vi "test Can Retry A Timed Out Future.vi"(8 "error in (no error)":errorcluster, 11 "TestCase in":refnum<class "Futures Tests.lvclass">) -> (0 "error out":errorcluster, 3 "TestCase out":refnum<class "Futures Tests.lvclass">)   [LabVIEW 2017, in "Futures Tests.lvclass"]
uses:
  Futures Tests.lvclass
  <vilib>/addons/_JKI Toolkits/VI Tester/TestCase.llb/TestCase.lvclass
  Futures/Futures.lvlib
  Futures/Future/Future.lvclass
  Futures/Promise/Promise.lvclass
  C:/Program Files (x86)/National Instruments/LabVIEW 2017/vi.lib/addons/_JKI Toolkits/VI Tester/TestCase.llb/TestCase.lvclass
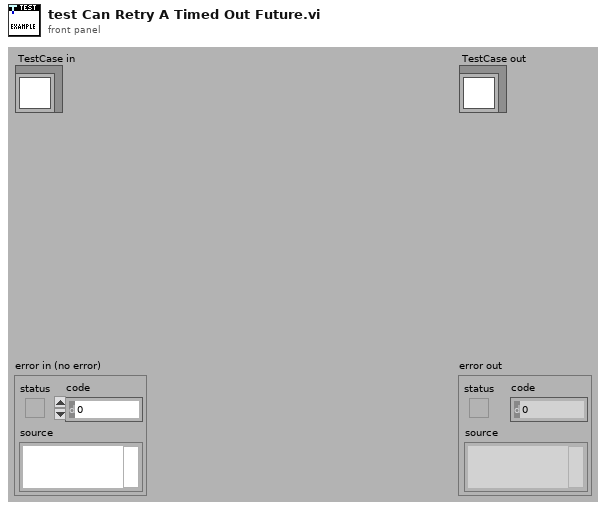
[diagram p1: front panel]
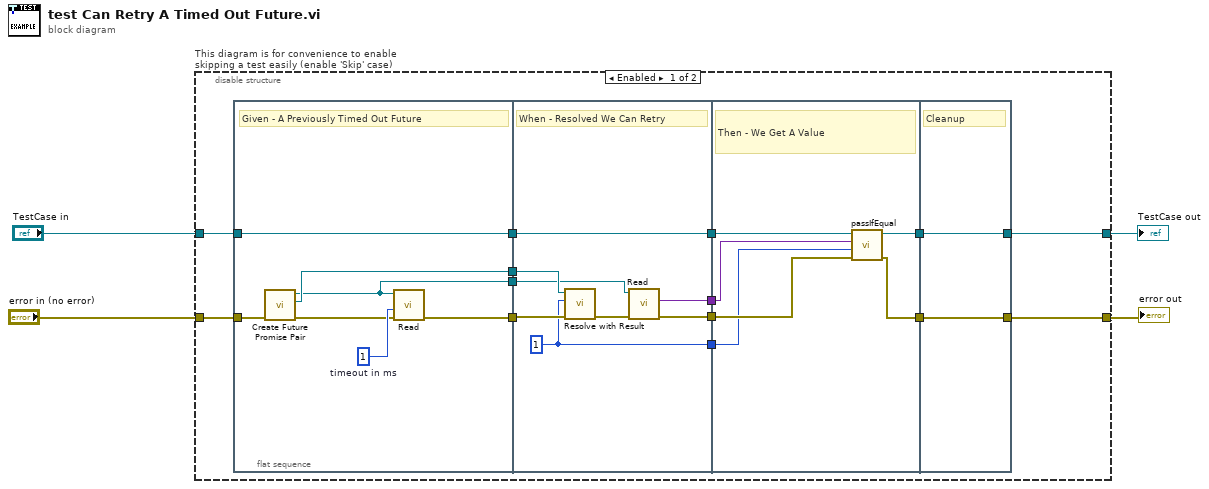
[diagram p0: block diagram]
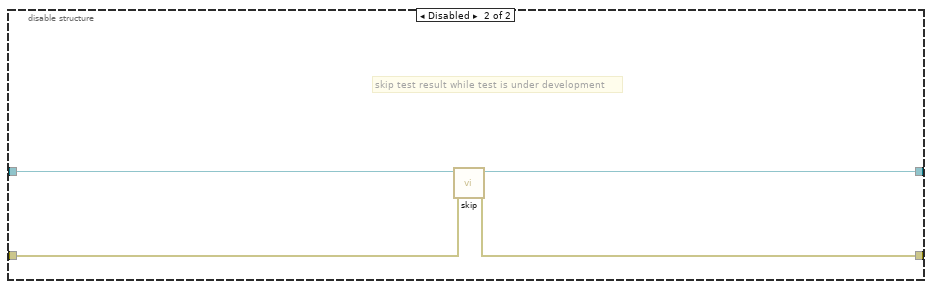
[diagram p2: hidden frame]
diagram:
  n1 = disable-structure "This diagram is for convenience to enable skipping a test easily (enable 'Skip' case)" shown="Enabled" {
    disable-tunnel: "TestCase in" -> [w14 w45]
    disable-tunnel: [w12 w43] -> w1
    disable-tunnel: [w11 w44] -> w3
    disable-tunnel: "error in (no error)" -> [w13 w42]
    frame Enabled {
      n2 = flat-sequence {
        tunnel: w13 -> [w24]
        tunnel: w14 -> [w25]
        tunnel: [w25] -> w18
        tunnel: [w21] -> w10
        tunnel: [w20] -> w9
        tunnel: [w19] -> w8
        tunnel: [w33] -> w17
        tunnel: w18 -> [w33]
        tunnel: w10 -> [w32]
        tunnel: w9 -> [w30]
        tunnel: w8 -> [w29]
        tunnel: [w28] -> w7
        tunnel: [w27] -> w6
        tunnel: [w26] -> w5
        tunnel: [w38] -> w16
        tunnel: [w37] -> w15
        tunnel: w17 -> [w39]
        tunnel: w7 -> [w36]
        tunnel: w6 -> [w35]
        tunnel: w5 -> [w34]
        tunnel: [w40] -> w11
        tunnel: [w41] -> w12
        tunnel: w16 -> [w41]
        tunnel: w15 -> [w40]
        frame #0 {
          w23 = 1  # timeout in ms
          # "Given - A Previously Timed Out Future"
          n3 = call "Create Future Promise Pair.vi"("error in (no error)"=w24) -> ("error out"=w22:errorcluster, "Promise out"=w20:refnum<class "Promise.lvclass">, "Future out"=w19:refnum<class "Future.lvclass">)  [unwired: 8 in]
          n4 = call "Read.vi"("error in (no error)"=w22, "timeout in ms (60 sec)"=w23, "Future in"=w19) -> ("error out"=w21:errorcluster)  [unwired: 5 in, 3 out]
        }
        frame #1 {
          w26 = 1
          # "When - Resolved We Can Retry"
          n5 = call "Resolve with Result.vi"("error in (no error)"=w32, "Result"=w26, "Promise in"=w30) -> ("error out"=w31:errorcluster)  [unwired: 8 in]
          n6 = call "Read.vi"("error in (no error)"=w31, "Future in"=w29) -> ("error out"=w28:errorcluster, "Result value"=w27:variant)  [unwired: 6 in, 2 out]
        }
        frame #2 {
          # "Then - We Get A Value"
          n7 = call-dynamic "passIfEqual.vi"("error in (no error)"=w36, "y"=w34, "x"=w35, "TestCase in"=w39) -> ("error out"=w37:errorcluster, "TestCase out"=w38:refnum<class "Futures Tests.lvclass">)  [unwired: 6 in]
        }
        frame #3 {
          # "Cleanup"
        }
      }
    }
    frame Disabled {
      # "skip test result while test is under development"
      n8 = call <vilib>:"skip.vi"("error in (no error)"=w42, "TestCase in"=w45) -> ("error out"=w44:errorcluster, "TestCase out"=w43:refnum<class "Futures Tests.lvclass">)  [unwired: 8 in]
    }
  }
  "error out" <- w3
  "TestCase out" <- w1
